vi "XY Graph Get Plot Names & Number.vi"(8 "error in (no error)":errorcluster, 11 "XYGraph in":T1) -> (0 "error out":errorcluster, 1 "# Plots":i32, 2 "Plot Names":string[](array[string]), 3 "XYGraph out":T1, 4 "Empty Plots?":bool[](array[boolean]), 5 "Graph Name":string)   [LabVIEW 2021, in "XY Graph Add-Ons.lvlib"]
uses:
  XY Graph Refnum.ctl
  XY Graph Add-Ons.lvlib
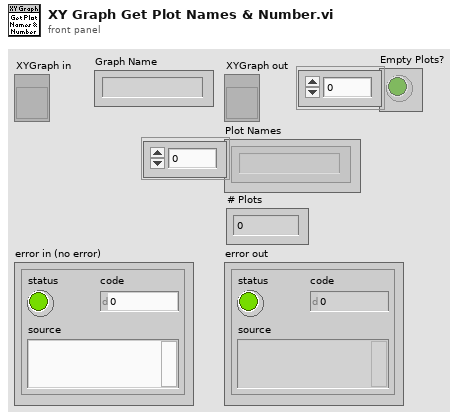
[diagram p1: front panel]
types:
  T1 = typedef "XY Graph Add-Ons.lvlib/XY Graph Refnum.ctl" = refnum<vi>
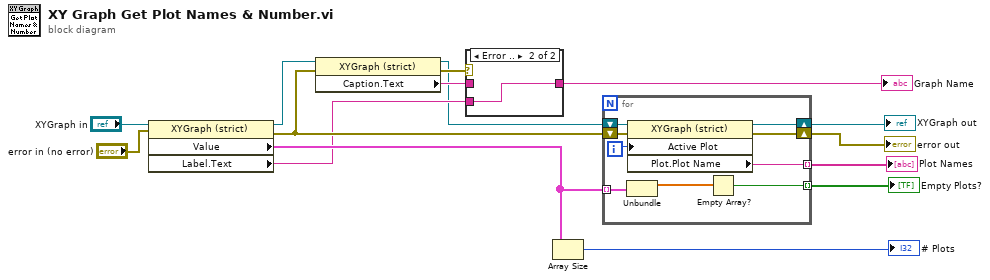
[diagram p0: block diagram]
diagram:
  n1 = property class="XYGraph (strict)"(reference="XYGraph in", error in="error in (no error)") -> (reference out=w6:T1, error out=w7:errorcluster, "Value"=w9:cluster{"X Array":dbl[], "Y Array":dbl[]}[], "Label.Text"=w2:string)
  n2 = property class="XYGraph (strict)"(reference=w6, error in=w7) -> (reference out=w1:T1, error out=w5:errorcluster, "Caption.Text"=w4:string)
  n3 = case shown="Error .." w5 {
    tunnel: w4 -> [w16 _]
    tunnel: [w16 w17] -> w3
    tunnel: w2 -> [_ w17]
    frame No Error {
    }
    frame Error {
    }
  }
  "Graph Name" <- w3
  n4 = Array Size(array=w9) -> (size(s)=→"# Plots":i32)
  n5 = for {
    shift-right: [w25] -> w14
    shift-left: w1 -> [w26]
    shift-right: [w21] -> w15
    shift-left: w7 -> [w24]
    tunnel: [w22] -> w10 mode=indexing
    tunnel: w9 -> [w20] mode=indexing
    tunnel: [w18] -> w8 mode=indexing
    i -> [w23]
    n6 = Unbundle(w20) -> ("X Array"=w19:dbl[])  [unwired: 1 out]
    n7 = property class="XYGraph (strict)"(reference=w26, error in=w24, "Active Plot"=w23) -> (reference out=w25:T1, error out=w21:errorcluster, "Plot.Plot Name"=w22:string)
    n8 = Empty Array?(array=w19) -> (empty?=w18:bool)
  }
  "error out" <- w15
  "XYGraph out" <- w14
  "Plot Names" <- w10
  "Empty Plots?" <- w8
